vi "unpack.vi"(11 "TCP Pack":string="\u0000resp      啊手动阀手动阀") -> (2 "tcp-message-type":T1=enum."resp", 3 "String":string="啊手动阀手动阀")   [LabVIEW 2020, in "CSM-TCP-Router.lvlib"]
uses:
  CSM-TCP-Router.lvlib
  typedef/tcp-msg type.ctl
  <userlib>/_NEVSTOP/Communicable State Machine(CSM)/Communicable State Machine.lvlib
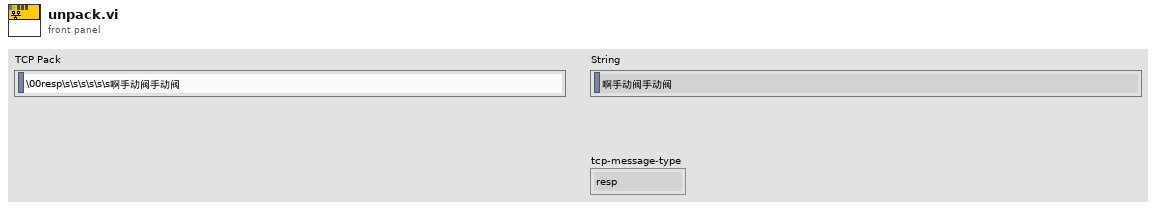
[diagram p1: front panel]
types:
  T1 = typedef "CSM-TCP-Router.lvlib/tcp-msg type.ctl" = enum16{"info", "error", "cmd", "resp", "async-resp", "status", "interrupt"}
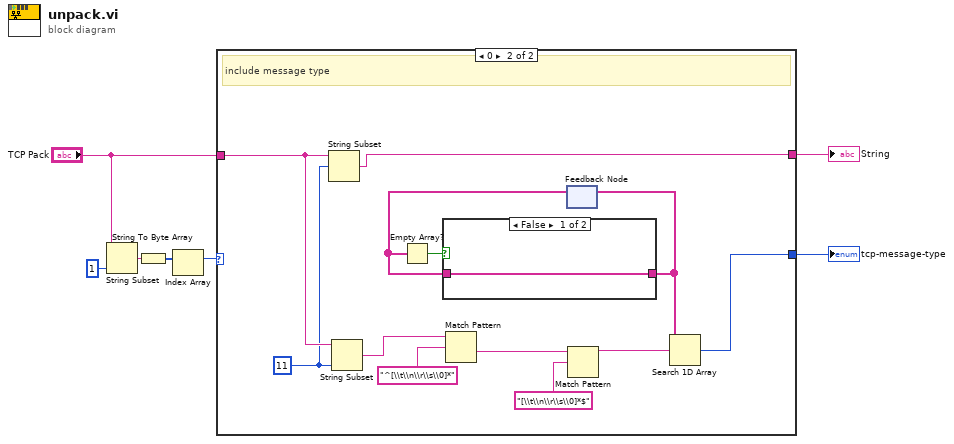
[diagram p0: block diagram]
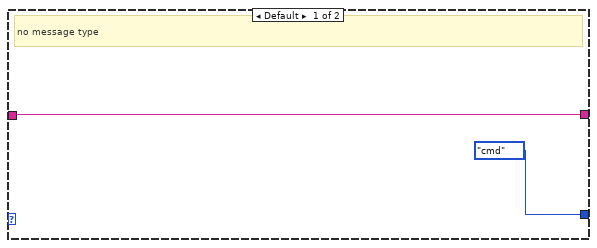
[diagram p2: hidden frame]
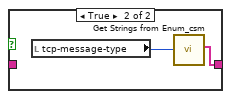
[diagram p3: hidden frame]
diagram:
  n1 = String Subset(string="TCP Pack", length (rest)=1 ("length (rest)")) -> (substring=w6:string)  [unwired: 1 in]
  n2 = String To Byte Array(string=w6) -> (unsigned byte array=w5:u8[])
  n3 = Index Array(array=w5) -> (element=w4:u8)  [unwired: 1 in]
  n4 = case shown="0" w4 {
    tunnel: "TCP Pack" -> [w9 w21]
    tunnel: [w9 w19] -> w2
    tunnel: [tcp-msg_type."cmd" ("tcp-message-type") w18] -> w1
    frame Default {
      # "no message type"
    }
    frame 0 {
      w20 = 11 ("length (rest)")
      # "include message type"
      n5 = String Subset(string=w21, offset (0)=w20) -> (substring=w19:string)  [unwired: 1 in]
      n6 = String Subset(string=w21, length (rest)=w20) -> (substring=w14:string)  [unwired: 1 in]
      n7 = Match Pattern(string=w14, regular expression="^[\\t\\n\\r\\s\\0]*") -> (after substring=w15:string)  [unwired: 1 in, 3 out]
      n8 = feedback #1() -> (w10:string[])  [unwired: 1 in]
      n9 = Empty Array?(array=w10) -> (empty?=w11:bool)
      n10 = case shown="False" w11 {
        tunnel: [w22 w23] -> w12
        tunnel: w10 -> [w22 _]
        frame False {
        }
        frame True {
          n11 = local read "tcp-message-type"() -> (w24:T1)
          n12 = call <userlib>:"Get Strings from Enum_csm.vi"("Enum"=w24) -> ("Enum Strings"=w23:string[])  [unwired: 7 in, 3 out]
        }
      }
      n13 = feedback-in #1(w12) -> ()
      n14 = Match Pattern(string=w15, regular expression="[\\t\\n\\r\\s\\0]*$") -> (before substring=w13:string)  [unwired: 1 in, 3 out]
      n15 = Search 1D Array(1D array=w12, element=w13) -> (index of element=w18:i32)  [unwired: 1 in]
    }
  }
  "String" <- w2
  "tcp-message-type" <- w1
